vi "PI_GCS2_Sample_Application_1_Controller.vi"() -> ()   [LabVIEW 2026]
doc: "This VI demonstrates how to initialize a PI GCS2 system and how to query the help answer. \nThe diagram shows how to combine the driver VIs for these tasks. \n\nWarning: Before running this VI, modify the interface settings on the block diagram to reflect your configuration. The predefined settings provided with the VI probably do not match your system."
uses:
  Low Level/Communication/Interface Settings.ctl
panel:
  out "Help string":string
  in  "stop":bool
  in  "error in":errorcluster
  out "Running":bool caption="Configuration_Setup.vi is running"
  out "error out":errorcluster
  out "Conn. Axis":string[](array[string])
  out "Identification":string
  # "This VI demonstrates how to initialize a PI GCS2 system and how to query the help answer. \nThe diagram shows how to combine the driver VIs for these tasks. \n\nWarning: Before running this VI, modify the interface settings on the block diagram to reflect your configuration. The predefined \n                 settings provided with the VI probably do not match your system."
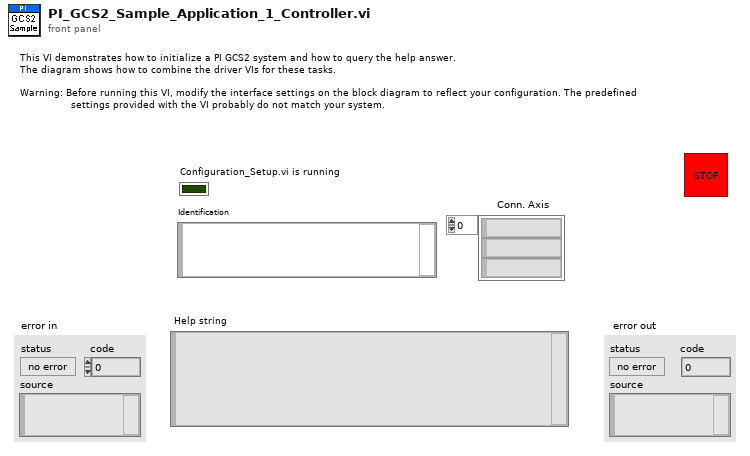
[diagram p1: front panel]
types:
  T1 = typedef "Interface Settings.ctl" = cluster{"Interface":u16, "Timeout":u32, "RS232 settings":cluster{"Portnumber":u8, "Baudrate":u16}, "TCP/IP settings":cluster{"Host address/name":string, "Port":i32, "Board":i32, "TCP/IP Search?":bool}, "USB settings":cluster{"S/N":string, "USB Search?":bool}, "DaisyChain settings":cluster{"Register DC":bool, "DaisyChain Search?":bool, "Device ID":i32}, "DLL for Device":u16}
  T2 = enum16{"Do not reference", "Reference switch", "Negative limit switch", "Positive limit switch"}[]
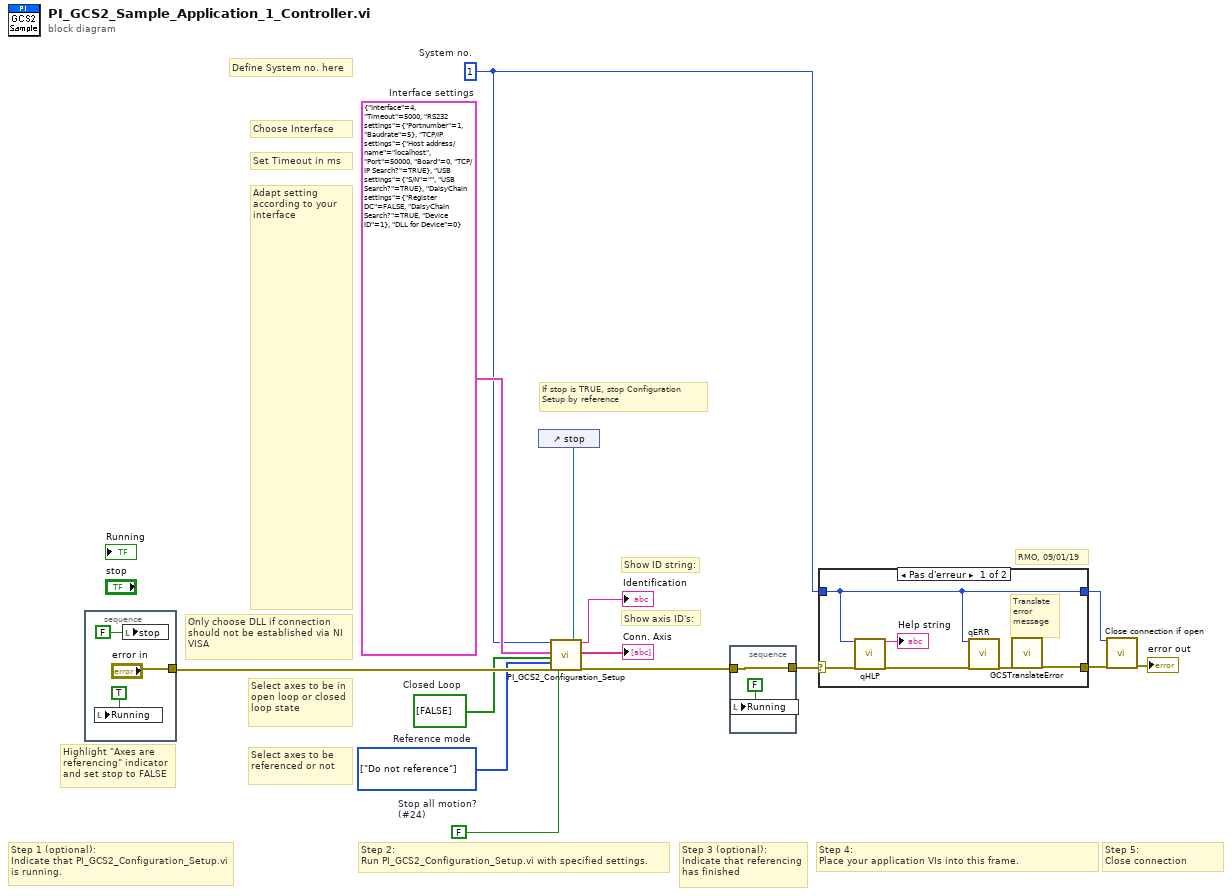
[diagram p0: block diagram]
diagram:
  w3 = T1 {"Interface"=4, "Timeout"=5000, "RS232 settings"={"Portnumber"=1, "Baudrate"=5}, "TCP/IP settings"={"Host address/name"="localhost", "Port"=50000, "Board"=0, "TCP/IP Search?"=TRUE}, "USB settings"={"S/N"="", "USB Search?"=TRUE}, "DaisyChain settings"={"Register DC"=FALSE, "DaisyChain Search?"=TRUE, "Device ID"=1}, "DLL for Device"=0}  # Interface settings
  w4 = FALSE  # Stop all motion? (#24)
  w5 = T2 [enum."Do not reference"] items=["Do not reference", "Reference switch", "Negative limit switch", "Positive limit switch"]  # Reference mode
  w6 = bool[] [FALSE]  # Closed Loop
  w2 = 1  # System no.
  # "Step 5:\nClose connection"
  # "Define System no. here"
  # "Select axes to be referenced or not"
  # "Select axes to be in open loop or closed loop state"
  # "Adapt setting according to your interface"
  # "Set Timeout in ms"
  # "Choose Interface"
  # "Only choose DLL if connection should not be established via NI VISA"
  # "If stop is TRUE, stop Configuration\nSetup by reference"
  # "Step 4: \nPlace your application VIs into this frame."
  # "RMO, 09/01/19"
  # "Step 3 (optional): \nIndicate that referencing has finished"
  # "Step 2: \nRun PI_GCS2_Configuration_Setup.vi with specified settings."
  # "Step 1 (optional): \nIndicate that PI_GCS2_Configuration_Setup.vi is running."
  # "Highlight \"Axes are\nreferencing\" indicator\nand set stop to FALSE"
  # "Show axis ID's:"
  # "Show ID string:"
  n1 = stacked-sequence {
    tunnel: ["error in"] -> w11
    frame #0 {
      n2 = local write "Running"(TRUE ("Running")) -> ()
      n3 = local write "stop"(FALSE ("stop")) -> ()
    }
  }
  n4 = control-ref of="stop"() -> (w12:refnum<vi>)
  n5 = call "PI_GCS2_Configuration_Setup.vi"("System no."=w2, "Interface settings"=w3, "Closed Loop"=w6, "Reference mode"=w5, "error in"=w11, "Stop all motion?"=w4, "Stop refnum"=w12) -> ("Identification"=→"Identification":string, "Conn. Axis"=→"Conn. Axis":string[], "error out"=w10:errorcluster)  [unwired: 1 in, 9 out]
  n6 = stacked-sequence {
    tunnel: w10 -> [w18]
    tunnel: [w18] -> w9
    frame #0 {
      n7 = local write "Running"(FALSE ("Running")) -> ()
    }
  }
  n8 = case shown="Pas d'erreur" w9 {
    selector: w9 -> [w23 w27]
    tunnel: [w25 w27] -> w13
    tunnel: w2 -> [w20 w26]
    tunnel: [w20 w26] -> w1
    frame No Error {
      # "Translate\nerror \nmessage"
      n9 = call "qHLP.vi"("System no."=w20, "error in"=w23) -> ("Help string"=→"Help string":string, "error out"=w22:errorcluster)  [unwired: 16 out]
      n10 = call "qERR.vi"("System no."=w20, "error in"=w22) -> ("error out"=w24:errorcluster)  [unwired: 17 out]
      n11 = call "GCSTranslateError.vi"("error in"=w24) -> ("error out"=w25:errorcluster)  [unwired: 18 out]
    }
    frame Error {
      # "Error during initialization"
    }
  }
  n12 = call "Close connection if open.vi"("System no."=w1, "error in"=w13) -> ("error out"=→"error out":errorcluster)  [unwired: 1 in, 16 out]
